vi "Login Dialog.vi"(11 "Authentication in":refnum<class "Authentication.lvclass">) -> (2 "Authenticated?":bool, 3 "Username Out":string="User 1")   [LabVIEW 2016, in "Authentication.lvclass"]
uses:
  Authentication.lvclass
panel:
  out "Message":string
  in  "Cancel":bool
  in  "Login":bool
  in  "Password":string
  in  "Username":string
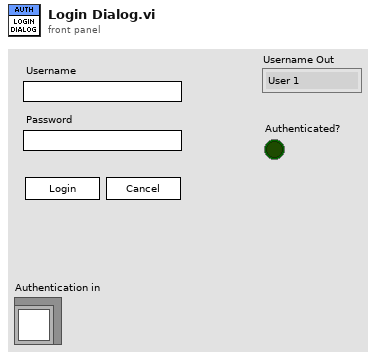
[diagram p1: front panel]
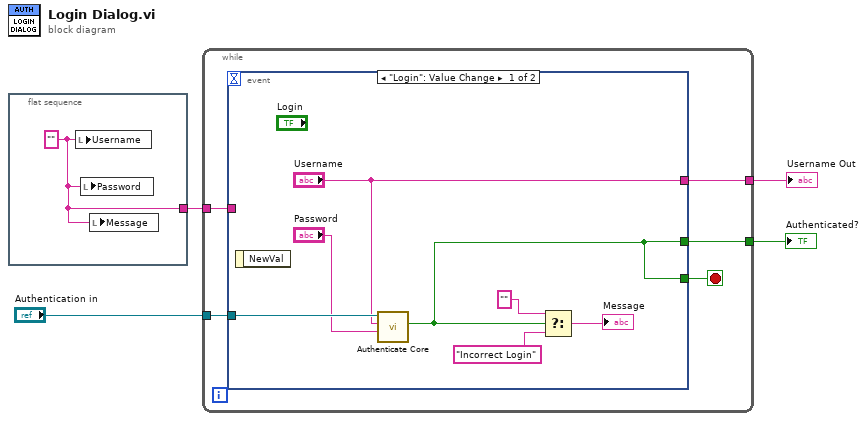
[diagram p0: block diagram]
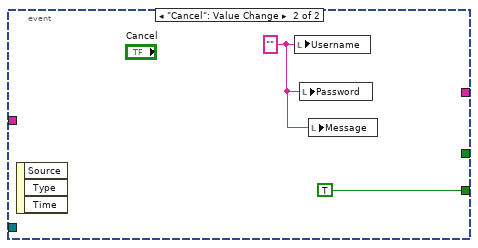
[diagram p2: hidden frame]
diagram:
  n1 = flat-sequence {
    tunnel: [w5] -> w2
    frame #0 {
      w5 = "" ("Username")
      n2 = local write "Username"(w5) -> ()
      n3 = local write "Password"(w5) -> ()
      n4 = local write "Message"(w5) -> ()
    }
  }
  n5 = while {
    tunnel: [w9] -> w3
    tunnel: w2 -> [w8]
    tunnel: [w10] -> w4
    tunnel: "Authentication in" -> [w6]
    stop <- w7 stop-if-true
    n6 = event shown="[0] \"Login\": Value Change" {
      selector: _ -> [_ _]
      dyn-events: _ -> [_ _]
      timeout: _ -> [_ _]
      tunnel: ["Username" _] -> w10
      tunnel: [w11 _] -> w9
      tunnel: w8 -> [_ _]
      tunnel: [w11 TRUE] -> w7
      tunnel: w6 -> [w14 _]
      event "Login": Value Change {
        n7 = event-data() -> ()  [unwired: 1 in, 1 out]
        n8 = call-dynamic "Authenticate Core.vi"("Password"="Password", "Username"="Username", "Authentication in"=w14) -> ("Authenticated?"=w11:bool)  [unwired: 6 in, 2 out]
        n9 = Select(t="", s=w11, f="Incorrect Login") -> (s? t:f=→"Message":string)
      }
      event "Cancel": Value Change {
        w18 = "" ("Username")
        n10 = event-data() -> ()  [unwired: 1 in, 3 out]
        n11 = local write "Username"(w18) -> ()
        n12 = local write "Password"(w18) -> ()
        n13 = local write "Message"(w18) -> ()
      }
    }
  }
  "Username Out" <- w4
  "Authenticated?" <- w3
